vi "Initialize.vi"(8 "error in (no error)":errorcluster, 11 "string handler":refnum<class "String Handler.lvclass">) -> (0 "error out":errorcluster, 3 "dup string handler":refnum<class "String Handler.lvclass">)   [LabVIEW 2018, in "Logging.lvlib" / "String Handler.lvclass"]
uses:
  String Handler.lvclass
  String Handler.lvclass/String Handler.ctl
panel:
  # "Connector Pane"
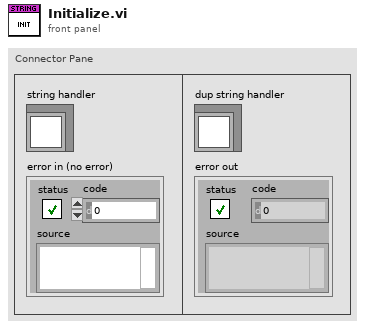
[diagram p1: front panel]
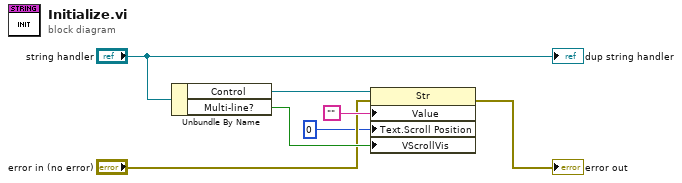
[diagram p0: block diagram]
diagram:
  n1 = Unbundle By Name("string handler") -> ("Control"=w7:refnum<vi>, "Multi-line?"=w5:bool)
  n2 = property class="Str"(reference=w7, error in="error in (no error)", "Value"="", "Text.Scroll Position"=u32 0, "VScrollVis"=w5) -> (error out=→"error out":errorcluster)  [unwired: 1 out]
  "dup string handler" <- "string handler"
